vi "Read Ghosts.vi"(8 "error in (no error)":errorcluster, 11 "Ghosts in":refnum<class "Ghosts.lvclass">) -> (0 "error out":errorcluster, 2 "Ghosts":T1, 3 "Ghosts out":refnum<class "Ghosts.lvclass">)   [LabVIEW 2016, in "PacManClasses.lvlib" / "Ghosts.lvclass"]
uses:
  Ghosts.lvclass
  Generic Controls/Ghosts.ctl
  Ghosts.lvclass/Ghosts.ctl
  PacManClasses.lvlib
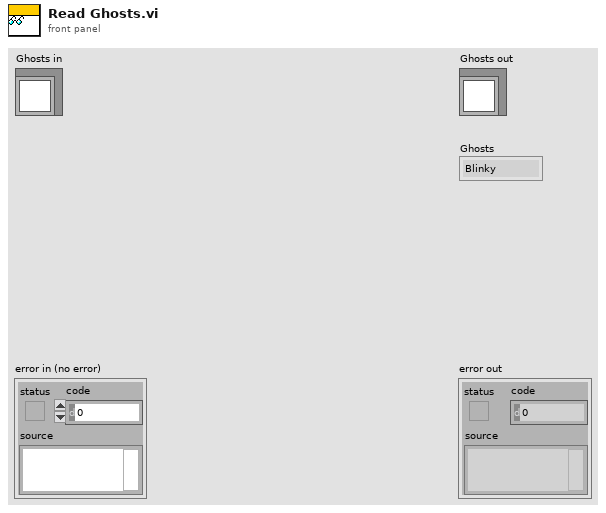
[diagram p1: front panel]
types:
  T1 = typedef "PacManClasses.lvlib/Ghosts.ctl" = enum16{"Blinky", "Pinky", "Inky", "Clyde"}
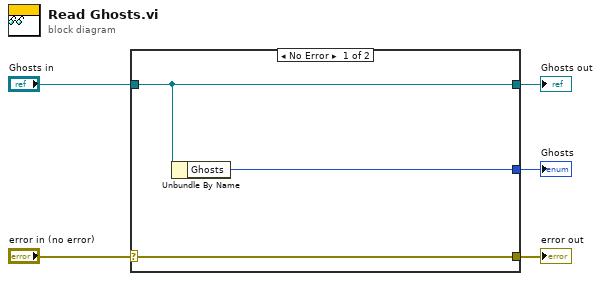
[diagram p0: block diagram]
diagram:
  n1 = case shown="No Error" "error in (no error)" {
    selector: "error in (no error)" -> [w8 w9]
    tunnel: [w8 w9] -> w4
    tunnel: [w7 w10] -> w2
    tunnel: "Ghosts in" -> [w7 w10]
    tunnel: [w6 _] -> w1
    frame No Error {
      n2 = Unbundle By Name(w7) -> ("Ghosts"=w6:T1)
    }
    frame Error {
    }
  }
  "error out" <- w4
  "Ghosts out" <- w2
  "Ghosts" <- w1
